vi "Item.vi"(8 "error in (no error)":errorcluster, 10 "Index":i32, 11 "ListImp in":refnum<class "ListImp.lvclass">) -> (0 "error out":errorcluster, 1 "Item":refnum<class>, 3 "ListImp out":refnum<class "ListImp.lvclass">)   [LabVIEW 2013, in "LapDog.Collections.v_.Lists.lvlib" / "ListImp.lvclass"]
doc: "Returns a copy of an item from the list at the given Index. An Index of -1 returns the last item in the list. If no item exists at the given Index error 510201 is returned."
uses:
  ListImp.lvclass
  LapDog.Collections.Common/LapDog.Collections.v_.Common.lvlib
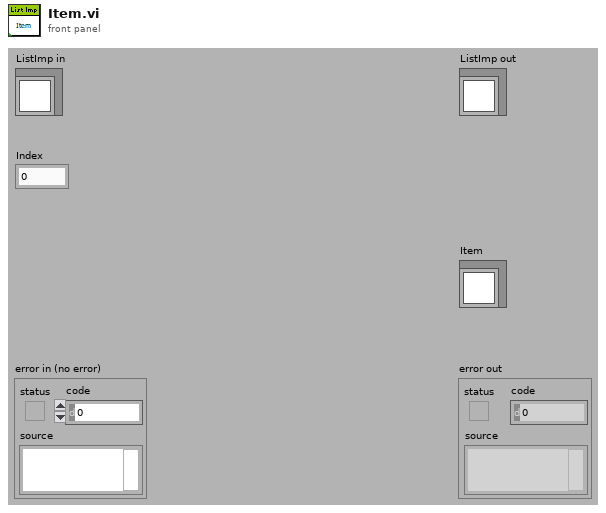
[diagram p1: front panel]
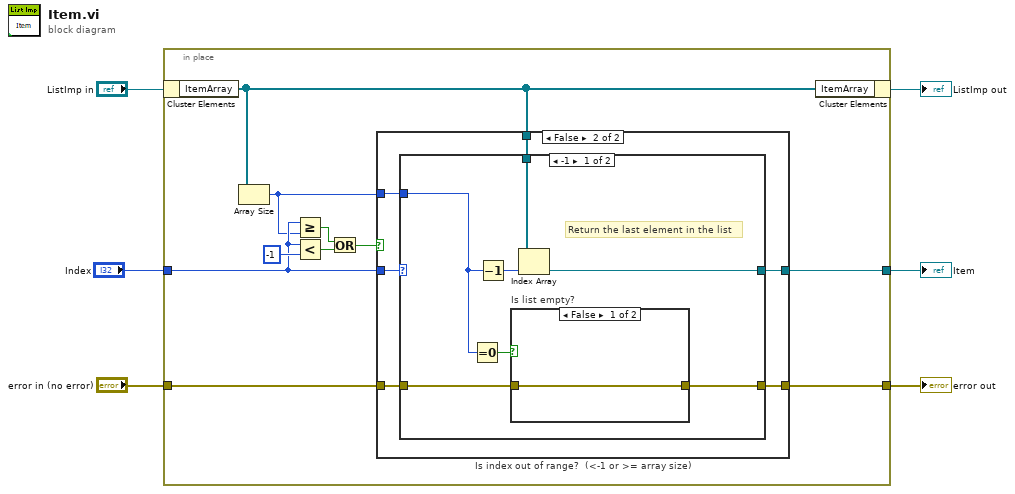
[diagram p0: block diagram]
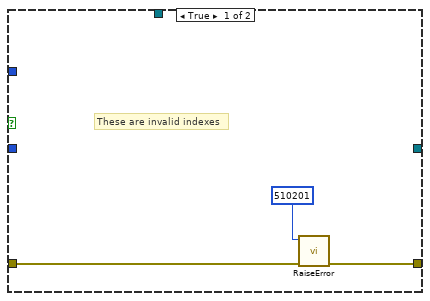
[diagram p2: hidden frame]
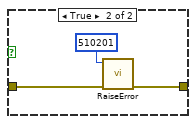
[diagram p3: hidden frame]
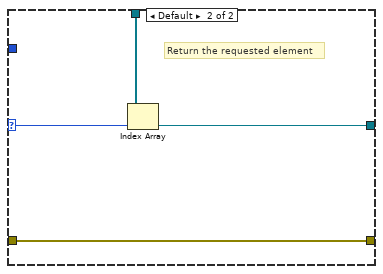
[diagram p4: hidden frame]
diagram:
  n1 = in-place {
    in-place-border: [w16] -> w6
    in-place-border: "error in (no error)" -> [w15]
    in-place-border: [w14] -> w4
    in-place-border: "Index" -> [w8]
    n2 = in-place-cluster #1("ListImp in") -> ("ItemArray"=w13:refnum<class>[])
    n3 = Array Size(array=w13) -> (size(s)=w7:i32)
    n4 = Greater Or Equal?(x=w8, y=w7) -> (x >= y?=w10:bool)
    n5 = Less?(x=w8, y=-1) -> (x < y?=w11:bool)
    n6 = Or(x=w10, y=w11) -> (x .or. y?=w9:bool)
    n7 = case "Is index out of range?  (<-1 or >= array size)" shown="False" w9 {
      tunnel: [_ w25] -> w16
      tunnel: w13 -> [_ w24]
      tunnel: w15 -> [w19 w21]
      tunnel: [w18 w20] -> w14
      tunnel: w8 -> [_ w23]
      tunnel: w7 -> [_ w22]
      frame True {
        # "These are invalid indexes"
        n8 = call "RaiseError.vi"("error in (no error)"=w19, "Error Code"=510201) -> ("error out"=w18:errorcluster)  [unwired: 9 in]
      }
      frame False {
        n9 = case shown="-1" w23 {
          selector: w23 -> [_ w38]
          tunnel: [w32 w40] -> w25
          tunnel: w24 -> [w31 w39]
          tunnel: w22 -> [w29 _]
          tunnel: w21 -> [w27 w37]
          tunnel: [w26 w37] -> w20
          frame -1 {
            # "Return the last element in the list"
            n10 = Equal To 0?(x=w29) -> (x = 0?=w28:bool)
            n11 = Decrement(x=w29) -> (x-1=w30:i32)
            n12 = case "Is list empty?" shown="False" w28 {
              tunnel: w27 -> [w33 w35]
              tunnel: [w33 w34] -> w26
              frame False {
              }
              frame True {
                n13 = call "RaiseError.vi"("error in (no error)"=w35, "Error Code"=510201) -> ("error out"=w34:errorcluster)  [unwired: 9 in]
              }
            }
            n14 = Index Array(array=w31, index=w30) -> (element=w32:refnum<class>)
          }
          frame Default {
            # "Return the requested element"
            n15 = Index Array(array=w39, index=w38) -> (element=w40:refnum<class>)
          }
        }
      }
    }
    n16 = in-place-cluster #1("ItemArray"=w13) -> (→"ListImp out":refnum<class "ListImp.lvclass">)
  }
  "error out" <- w4
  "Item" <- w6
